vi "Test Deserialize Null.vi"(8 "error in (no error)":errorcluster) -> (0 "error out":errorcluster)   [LabVIEW 2015]
uses:
  <vilib>/addons/_JKI Toolkits/Caraya/classes/Test/Test.lvclass
  src/JKI JSON Serialization.lvlib
  <vilib>/addons/_JKI Toolkits/Caraya/classes/Assert/Assert.lvclass
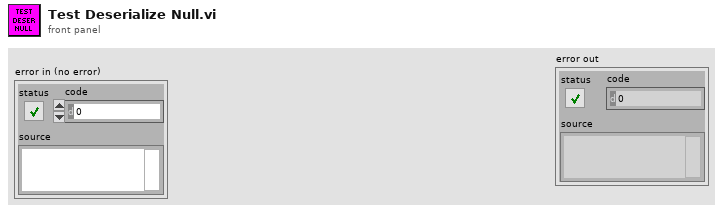
[diagram p1: front panel]
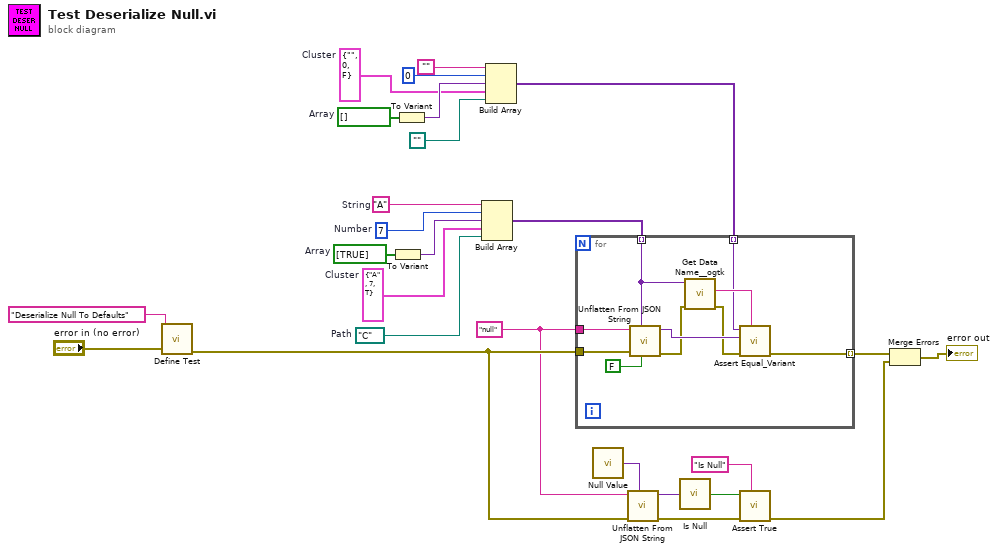
[diagram p0: block diagram]
diagram:
  w9 = cluster{"String":string, "Number":i32, bool} {"String"="", "Number"=0, FALSE}  # Cluster
  w14 = path "C:/"  # Path
  w16 = bool[] []  # Array
  w19 = cluster{"String":string, "Number":i32, bool} {"String"="A", "Number"=7, TRUE}  # Cluster
  w20 = bool[] [TRUE]  # Array
  w21 = 7  # Number
  w17 = "A"  # String
  w6 = "null" ("JSON String")
  n1 = call <vilib>:"Define Test.vi"("error in (no error)"="error in (no error)", "Label (VI Title)"="Deserialize Null To Defaults") -> ("error out"=w7:errorcluster)  [unwired: 9 in]
  n2 = To Variant(anything=w20) -> (Variant=w18:variant)
  n3 = To Variant(anything=w16) -> (Variant=w15:variant)
  n4 = Build Array(w17, w21, w18, w19, w14) -> (w22:variant[])
  n5 = Build Array("", 0 ("Number"), w15, w9, path "") -> (w12:variant[])
  n6 = for {
    tunnel: w6 -> [w36]
    tunnel: [w30] -> w23 mode=indexing
    tunnel: w7 -> [w29]
    tunnel: w22 -> [w28] mode=indexing
    tunnel: w12 -> [w27] mode=indexing
    n7 = call "Unflatten From JSON String.vi"("Nulls as Defaults (F)"=FALSE ("Nulls as Defaults (T)"), "Type and Defaults"=w28, "error in (no error)"=w29, "JSON String"=w36) -> ("error out"=w32:errorcluster, "Variant"=w34:variant)  [unwired: 6 in]
    n8 = call <userlib>:"Get Data Name__ogtk.vi"("error in (no error)"=w32, "Data"=w28) -> ("error out"=w31:errorcluster, "Data Name"=w33:string)  [unwired: 7 in, 1 out]
    n9 = call <vilib>:"Assert Equal_Variant.vi"("Label"=w33, "error in (no error)"=w31, "Y"=w34, "X"=w27) -> ("error out"=w30:errorcluster)  [unwired: 7 in]
  }
  n10 = call "Null Value.vi"() -> ("Null"=w1:variant)
  n11 = call "Unflatten From JSON String.vi"("Type and Defaults"=w1, "error in (no error)"=w7, "JSON String"=w6) -> ("error out"=w8:errorcluster, "Variant"=w5:variant)  [unwired: 7 in]
  n12 = call "Is Null.vi"("Deserialized JSON Data"=w5) -> ("Null?"=w4:bool)
  n13 = call <vilib>:"Assert True.vi"("Label"="Is Null", "error in (no error)"=w8, "True?"=w4) -> ("error out"=w3:errorcluster)  [unwired: 8 in]
  n14 = Merge Errors(w23, w3) -> (→"error out":errorcluster)
